vi "WaitForInit.vi"(8 "error in (no error)":errorcluster, 11 "Connection in":refnum<class "Connection.lvclass">) -> (0 "error out":errorcluster, 3 "Connection out":refnum<class "Connection.lvclass">)   [LabVIEW 2022 SP3, in "Connection.lvlib" / "Connection.lvclass"]
uses:
  Connection.lvclass
  C:/Program Files (x86)/National Instruments/LabVIEW 2022/vi.lib/ActorFramework/Actor/Actor.lvclass
  C:/Users/jakub/repos/gh/sw4sys/lv-tcp-server-sample/LoggingActor/Source/LoggingActor/LoggingActor/LoggingActor.lvclass
  Connection.lvclass/Connection.ctl
  <vilib>/ActorFramework/Actor/Actor.lvclass/Actor.ctl
  <vilib>/ActorFramework/Message Enqueuer/Message Enqueuer.lvclass/Message Enqueuer.ctl
  LoggingActor/Source/LoggingActor/LoggingActor/LoggingActor.lvclass/LoggingActor.ctl
  LoggingActor/Source/LoggingActor/LoggingActor/Read Logger.vi
  <vilib>/ActorFramework/Message Enqueuer/Init from Existing Queue.vi
  <vilib>/ActorFramework/Message Enqueuer/Enqueue.vi
  Connection Messages/WaitForInit Msg/WaitForInit Msg.lvclass
  C:/Program Files (x86)/National Instruments/LabVIEW 2022/vi.lib/ActorFramework/Message/Message.lvclass
  Connection Messages/Kill Msg/Kill Msg.lvclass
  <vilib>/ActorFramework/Message Priority Queue/Priority Enqueue.vi
  <vilib>/ActorFramework/Message Enqueuer/Message Enqueuer.lvclass
  Logger/Source/Logger/Logger.lvclass
  <vilib>/ActorFramework/Actor/Actor.lvclass
  C:/Users/jakub/repos/gh/sw4sys/lv-tcp-server-sample/TcpServerSample/Source/TcpServerSample/Connection/Connection/Connection.lvclass
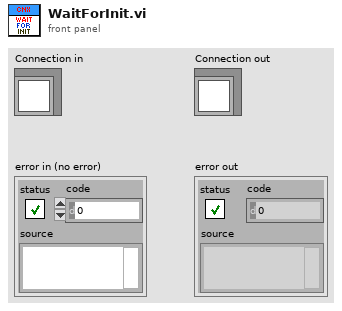
[diagram p1: front panel]
types:
  T1 = typedef "Connection.lvlib/Connection.lvclass/_State.ctl" = enum16{"WaitForInit", "Active", "Dying"}
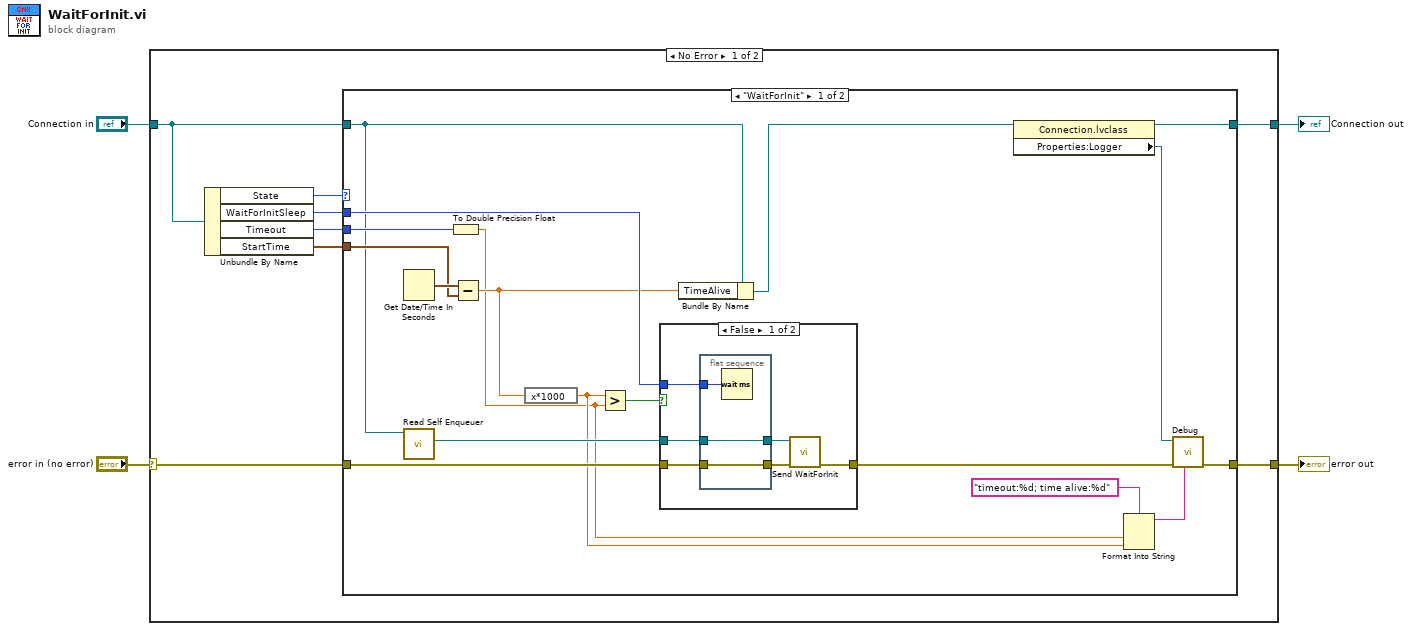
[diagram p0: block diagram]
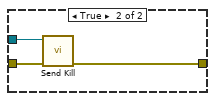
[diagram p2: hidden frame]
diagram:
  n1 = case shown="No Error" "error in (no error)" {
    selector: "error in (no error)" -> [w9 w46]
    tunnel: [w8 w46] -> w3
    tunnel: [w11 w45] -> w1
    tunnel: "Connection in" -> [w5 w45]
    frame No Error {
      n2 = Unbundle By Name(w5) -> ("State"=w6:T1, "WaitForInitSleep"=w7:u32, "Timeout"=w10:i32, "StartTime"=w12:timestamp)
      n3 = case shown="\"WaitForInit\"" w6 {
        tunnel: w12 -> [w29 _]
        tunnel: [w19 w44] -> w11
        tunnel: w10 -> [w27 _]
        tunnel: w9 -> [w26 w43]
        tunnel: [w20 w43] -> w8
        tunnel: w5 -> [w21 w44]
        tunnel: w7 -> [w22 _]
        frame "WaitForInit" {
          n4 = Get Date/Time In Seconds() -> (seconds since 1Jan1904=w30:timestamp)
          n5 = call <vilib>:"Read Self Enqueuer.vi"("Actor"=w21) -> ("Self Enqueuer"=w23:refnum<class "Message Enqueuer.lvclass">)  [unwired: 10 in]
          n6 = To Double Precision Float(number=w27) -> (double precision float=w13:dbl)
          n7 = Subtract(x=w30, y=w29) -> (x-y=w15:dbl)
          n8 = expression code="x*1000"(w15) -> (w14:dbl)
          n9 = Greater?(x=w14, y=w13) -> (0:w24:bool)
          n10 = case shown="False" w24 {
            tunnel: [w36 w42] -> w25
            tunnel: w26 -> [w34 w41]
            tunnel: w23 -> [w33 w40]
            tunnel: w22 -> [w35 _]
            frame False {
              n11 = flat-sequence {
                tunnel: w35 -> [w39]
                tunnel: w34 -> [w37]
                tunnel: w33 -> [w38]
                tunnel: [w38] -> w32
                tunnel: [w37] -> w31
                frame #0 {
                  n12 = Wait (ms)(milliseconds to wait=w39) -> ()  [unwired: 1 out]
                }
              }
              n13 = call "Send WaitForInit.vi"("error in (no error)"=w31, "Message Enqueuer"=w32) -> ("error out"=w36:errorcluster)  [unwired: 8 in, 1 out]
            }
            frame True {
              n14 = call "Send Kill.vi"("error in (no error)"=w41, "Message Enqueuer"=w40) -> ("error out"=w42:errorcluster)  [unwired: 8 in, 1 out]
            }
          }
          n15 = Bundle By Name(cluster=w21, "TimeAlive"=w15) -> (w28:refnum<class "Connection.lvclass">)
          n16 = property class="Connection.lvclass"(reference=w28) -> (reference out=w19:refnum<class "Connection.lvclass">, "Properties:Logger"=w18:refnum<class "Logger.lvclass">)  [unwired: 1 in, 1 out]
          n17 = Format Into String(format string="timeout:%d; time alive:%d", w13, w14) -> (resulting string=w16:string)  [unwired: 2 in, 1 out]
          n18 = call-dynamic "Debug.vi"("Message"=w16, "error in (no error)"=w25, "Logger in"=w18) -> ("error out"=w20:errorcluster)  [unwired: 5 in, 1 out]
        }
        frame Default {
        }
      }
    }
    frame Error {
    }
  }
  "error out" <- w3
  "Connection out" <- w1
